vi "DSP test 1.vi"() -> ()   [LabVIEW 2009, in "MicroDAQ.lvlib"]
uses:
  <instrlib>/MicroDAQ/MicroDAQ.lvlib
  <instrlib>/MicroDAQ/Channel/DSP/DSP.lvclass
panel:
  in  "Write enable":bool=TRUE
  out "Loop iteration duration [ms]":u32(graph)
  out "Write duration [ms]":u32(graph)
  out "Read duration [ms]":u32(graph)
  out "Start duration [ms]":u32
  in  "Rate [Hz]":dbl=10.0
  in  "Number of channels to read":i32=2
  in  "XCOS SIGNAL ID":i32=1
  in  "READ: Samples count":i32=1
  out "data out":dbl[][](array[numeric])
  in  "data in":sgl[](array[numeric])=[2.0, 3.0]
  in  "stop":bool
  in  "DSP binary path":path=path "C:/Program Files (x86)/National Instruments/LabVIEW 2014/instr.lib/MicroDAQ/Temp Tests/app1.out"
  # "DSP time diagnostic"
  # "DSP settings and data"
  # "TIME"
  # "Disable Write function to test Read function only."
  # "Czas wykonywania się funkcji DSP_read oraz DSP_write nie jest stał, periodycznie pojawiaja się czasy wykonania o 50% dłuższe niż czas oczekiwany. Do sprawdzenia czasów można wykorzystać \"DSP test 1.vi\"."
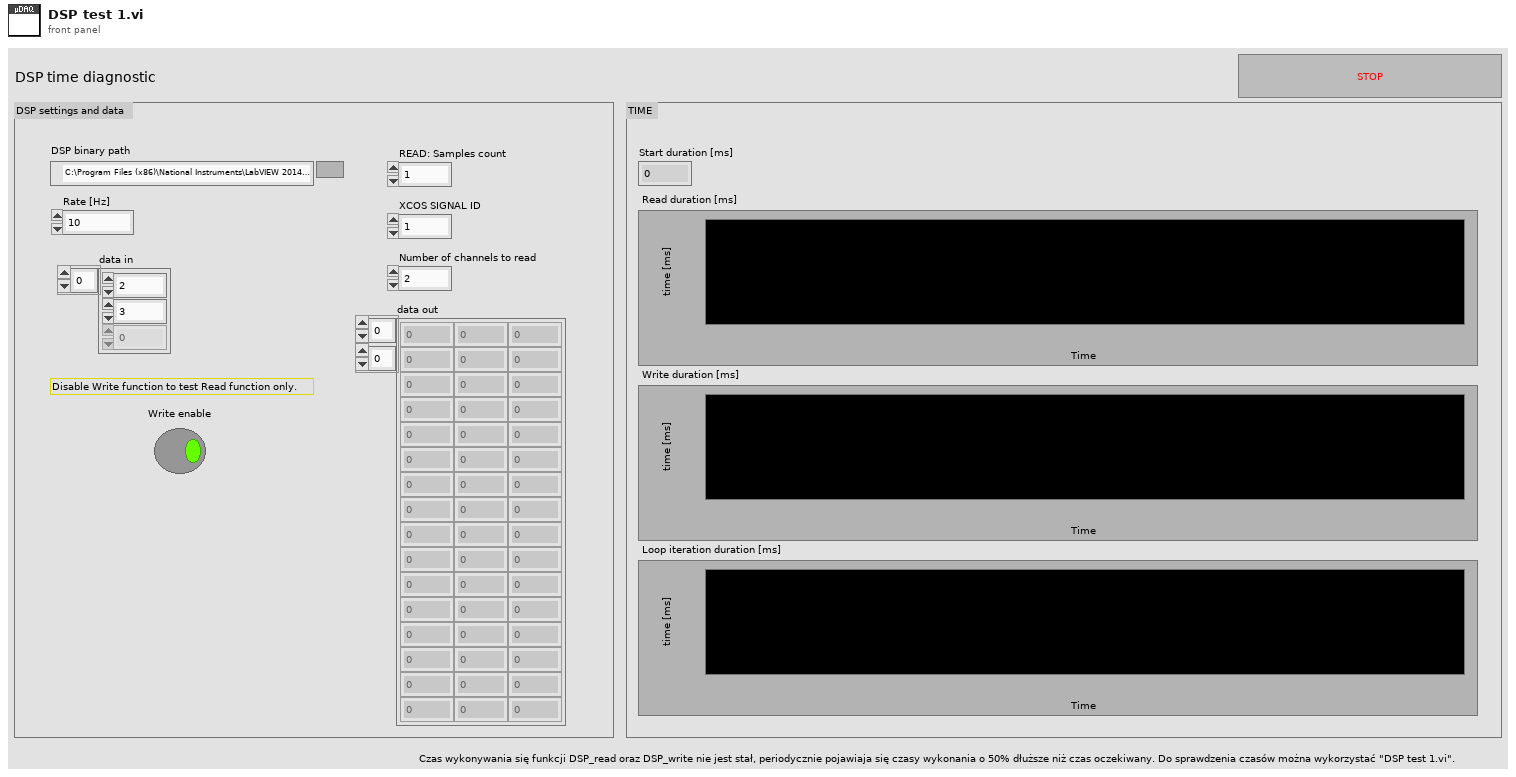
[diagram p1: front panel]
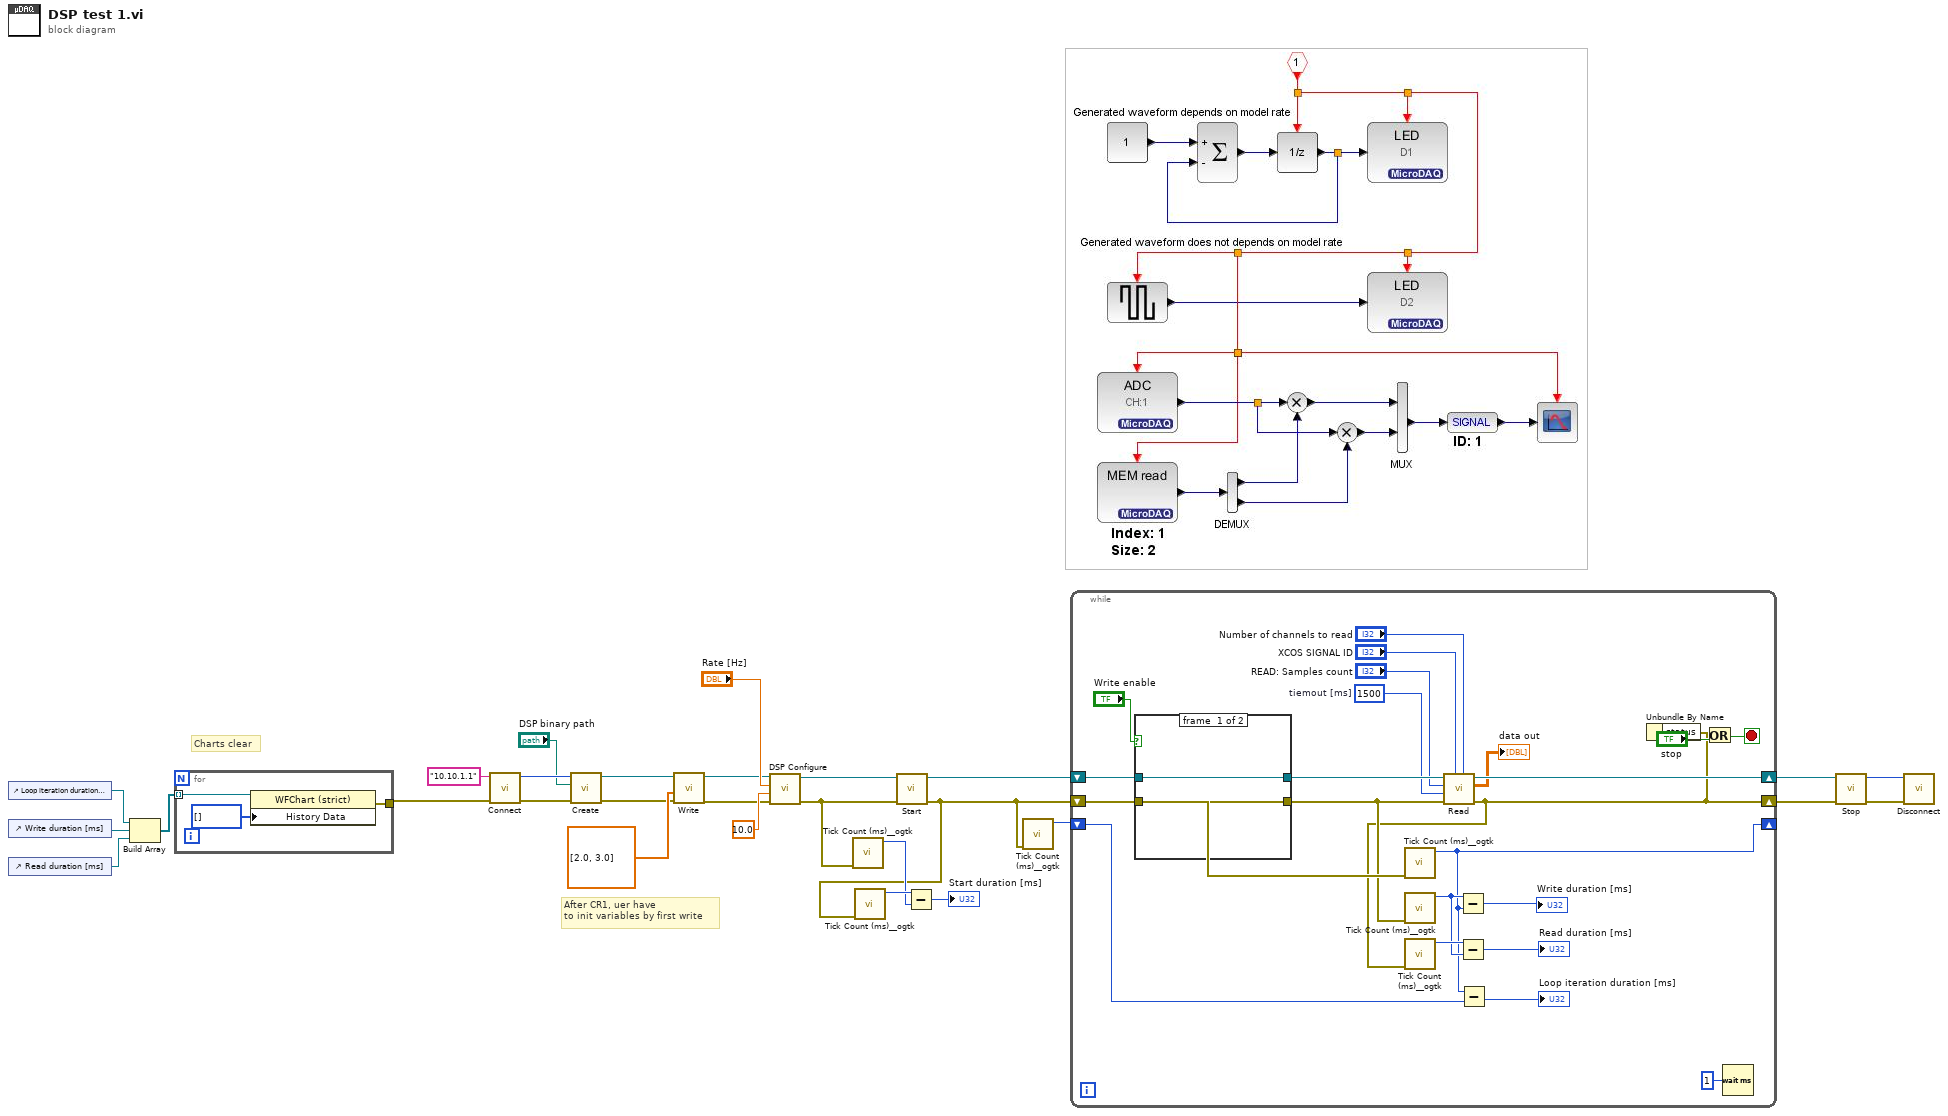
[diagram p0: block diagram]
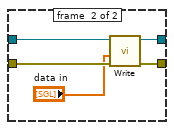
[diagram p2: hidden frame]
diagram:
  # "After CR1, uer have\nto init variables by first write"
  # "Charts clear"
  n1 = control-ref of="Loop iteration duration [ms]"() -> (w10:refnum<vi>)
  n2 = control-ref of="Write duration [ms]"() -> (w11:refnum<vi>)
  n3 = control-ref of="Read duration [ms]"() -> (w9:refnum<vi>)
  n4 = Build Array(w10, w11, w9) -> (w8:refnum<vi>[])
  n5 = for {
    tunnel: w8 -> [w31] mode=indexing
    tunnel: [w29] -> w6
    n6 = property class="WFChart (strict)"(reference=w31, "History Data"=u32[] []) -> (error out=w29:errorcluster)  [unwired: 1 in, 1 out]
  }
  n7 = call <instrlib>:"Connect.vi"("error in (no error)"=w6, "IP address"="10.10.1.1") -> ("error out"=w27:errorcluster, "connection ID"=w26:i32)  [unwired: 8 in]
  n8 = call <instrlib>:"Create.vi"("error in (no error)"=w27, "DSP binary path"="DSP binary path", "connection ID"=w26) -> ("error out"=w1:errorcluster, "MicroDAQ.lvlib:DSP.lvclass"=w4:refnum<class "DSP.lvclass">)  [unwired: 7 in]
  n9 = call <instrlib>:"Write.vi"("error in"=w1, "data"=sgl[] [2.0, 3.0] ("Init Values"), "MicroDAQ.lvlib:DSP.lvclass"=w4) -> ("error out"=w2:errorcluster, "MicroDAQ.lvlib:DSP.lvclass out"=w3:refnum<class "DSP.lvclass">)  [unwired: 7 in]
  n10 = call <instrlib>:"DSP Configure.vi"("error in"=w2, "duration [s]"=10.0, "Rate [Hz]"="Rate [Hz]", "MicroDAQ.lvlib:DSP.lvclass"=w3) -> ("error out"=w17:errorcluster, "MicroDAQ.lvlib:DSP.lvclass out"=w19:refnum<class "DSP.lvclass">)  [unwired: 6 in]
  n11 = call <userlib>:"Tick Count (ms)__ogtk.vi"("error in (no error)"=w17) -> ("millisecond timer value"=w15:u32)  [unwired: 9 in, 1 out]
  n12 = call-dynamic "Start.vi"("error in (no error)"=w17, "Task in"=w19) -> ("error out"=w12:errorcluster, "Task out"=w24:refnum<class "DSP.lvclass">)  [unwired: 8 in]
  n13 = call <userlib>:"Tick Count (ms)__ogtk.vi"("error in (no error)"=w12) -> ("millisecond timer value"=w16:u32)  [unwired: 9 in, 1 out]
  n14 = Subtract(x=w16, y=w15) -> (x-y=→"Start duration [ms]":u32)
  n15 = call <userlib>:"Tick Count (ms)__ogtk.vi"("error in (no error)"=w12) -> ("millisecond timer value"=w13:u32)  [unwired: 9 in, 1 out]
  n16 = while {
    shift-right: [w52] -> w22
    shift-left: w24 -> [w54]
    shift-right: [w41] -> w23
    shift-left: w12 -> [w43]
    shift-right: [w36] -> _
    shift-left: w13 -> [w35]
    stop <- w45 stop-if-true
    w48 = 1500  # tiemout [ms]
    n17 = case shown="True" "Write enable" {
      tunnel: w54 -> [w56 w61]
      tunnel: [w56 w60] -> w53
      tunnel: w43 -> [w55 w59]
      tunnel: [w55 w58] -> w42
      frame #0 {
      }
      frame #1 {
        n18 = call <instrlib>:"Write.vi"("error in"=w59, "data"="data in", "MicroDAQ.lvlib:DSP.lvclass"=w61) -> ("error out"=w58:errorcluster, "MicroDAQ.lvlib:DSP.lvclass out"=w60:refnum<class "DSP.lvclass">)  [unwired: 7 in]
      }
    }
    n19 = call <userlib>:"Tick Count (ms)__ogtk.vi"("error in (no error)"=w43) -> ("millisecond timer value"=w36:u32)  [unwired: 9 in, 1 out]
    n20 = call <userlib>:"Tick Count (ms)__ogtk.vi"("error in (no error)"=w42) -> ("millisecond timer value"=w39:u32)  [unwired: 9 in, 1 out]
    n21 = call <instrlib>:"Read.vi"("Number of channels to read"="Number of channels to read", "signal id"="XCOS SIGNAL ID", "error in"=w42, "tiemout [s]"=w48, "Samples count"="READ: Samples count", "MicroDAQ.lvlib:DSP.lvclass"=w53) -> ("error out"=w41:errorcluster, "data"=→"data out":dbl[][], "MicroDAQ.lvlib:DSP.lvclass out"=w52:refnum<class "DSP.lvclass">)  [unwired: 3 in]
    n22 = call <userlib>:"Tick Count (ms)__ogtk.vi"("error in (no error)"=w41) -> ("millisecond timer value"=w40:u32)  [unwired: 9 in, 1 out]
    n23 = Subtract(x=w39, y=w36) -> (x-y=→"Write duration [ms]":u32)
    n24 = Subtract(x=w40, y=w39) -> (x-y=→"Read duration [ms]":u32)
    n25 = Subtract(x=w36, y=w35) -> (x-y=→"Loop iteration duration [ms]":u32)
    n26 = Unbundle By Name(w41) -> ("status"=w32:bool)
    n27 = Or(x=w32, y="stop") -> (x .or. y?=w45:bool)
    n28 = Wait (ms)(milliseconds to wait=u32 1) -> ()  [unwired: 1 out]
  }
  n29 = call-dynamic "Stop.vi"("error in (no error)"=w23, "Task in"=w22) -> ("error out"=w21:errorcluster, "connection ID"=w20:i32)  [unwired: 8 in]
  n30 = call <instrlib>:"Disconnect.vi"("error in (no error)"=w21, "connection ID"=w20) -> ()  [unwired: 9 in, 1 out]
